vi "Backpropagation.vi"(8 "All Inputs":T2[](array[typedef]), 9 "Derrivatives":T2[](array[typedef]), 10 "Error":dbl[](array[numeric]), 11 "Neural Network In":refnum<class "Neural Network.lvclass">) -> (1 "Gradient Out":T1[](array[typedef]))   [LabVIEW 2015, in "Neural Network.lvclass"]
uses:
  Neural Network.lvclass
  Types/2D Array.ctl
  <vilib>/Analysis/NI_AALBase.lvlib
  <vilib>/Analysis/baseanly.llb/Real Outer Product.vi
  <vilib>/Analysis/Matrix/NI_Matrix.lvlib
  <vilib>/Analysis/Matrix/Numeric/Conversions/Matrix To Array - RM.vi
  Types/1D Array.ctl
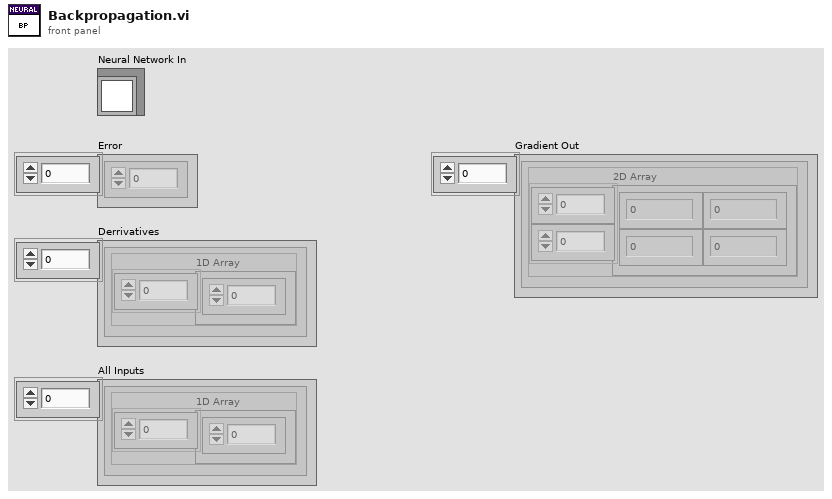
[diagram p1: front panel]
types:
  T1 = typedef "Neural Network.lvclass/2D Array.ctl" = cluster{"2D Array":sgl[][]}
  T2 = typedef "Neural Network.lvclass/1D Array.ctl" = cluster{"1D Array":dbl[]}
  T3 = typedef "NI_Matrix.lvlib/RealMatrix.ctl" = dbl[][]
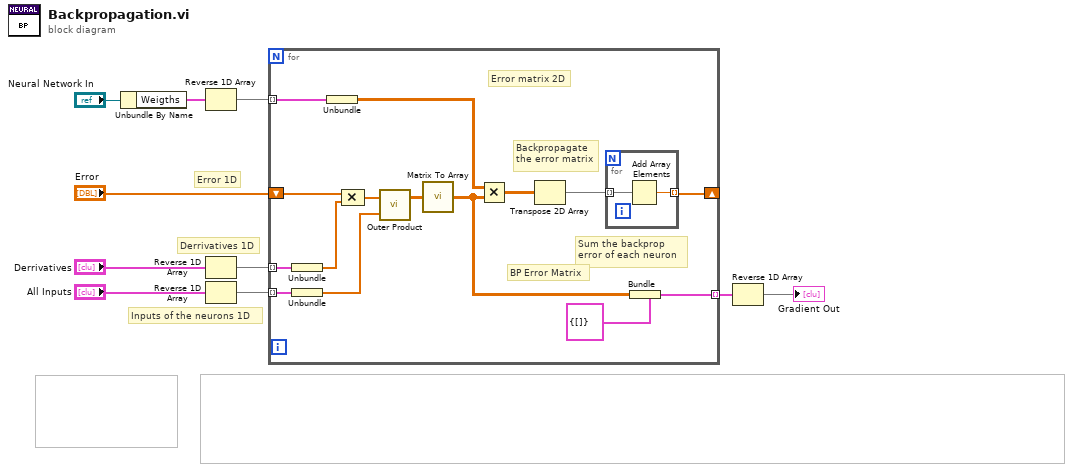
[diagram p0: block diagram]
diagram:
  # "Error 1D"
  # "Inputs of the neurons 1D"
  # "Derrivatives 1D"
  n1 = Unbundle By Name("Neural Network In") -> ("Weigths"=w1:T1[])
  n2 = Reverse 1D Array(array=w1) -> (reversed array=w9:T1[])
  n3 = Reverse 1D Array(array="Derrivatives") -> (reversed array=w7:T2[])
  n4 = Reverse 1D Array(array="All Inputs") -> (reversed array=w8:T2[])
  n5 = for {
    tunnel: w7 -> [w25] mode=indexing
    tunnel: w8 -> [w24] mode=indexing
    tunnel: w9 -> [w18] mode=indexing
    shift-right: [w22] -> _
    shift-left: "Error" -> [w20]
    tunnel: [w21] -> w10 mode=indexing
    # "BP Error Matrix"
    # "Sum the backprop\nerror of each neuron"
    # "Backpropagate\nthe error matrix"
    # "Error matrix 2D"
    n6 = Unbundle(w25) -> ("1D Array"=w23:dbl[])
    n7 = Unbundle(w24) -> ("1D Array"=w15:dbl[])
    n8 = Unbundle(w18) -> ("2D Array"=w13:sgl[][])
    n9 = Compound Arithmetic op=MULTIPLY(w20, w23) -> (w16:dbl[])
    n10 = call-poly <vilib>:"Outer Product.vi"("Y Vector"=w15, "X Vector"=w16) -> ("Outer Product"=w14:T3)  [unwired: 1 out]
    n11 = call-poly <vilib>:"Matrix To Array.vi"("Real Matrix"=w14) -> ("Real 2D Array"=w11:dbl[][])
    n12 = Multiply ("Multiply.vi")(x=w13, y=w11) -> (x*y=w12:dbl[][])
    n13 = Transpose 2D Array(2D array=w12) -> (transposed array=w17:dbl[][])
    n14 = for {
      tunnel: w17 -> [w27] mode=indexing
      tunnel: [w26] -> w22 mode=indexing
      n15 = Add Array Elements(numeric array=w27) -> (sum=w26:dbl)
    }
    n16 = Bundle(cluster=T1 {"2D Array"=[]}, "2D Array"=w11) -> (w21:T1)
  }
  n17 = Reverse 1D Array(array=w10) -> (reversed array=→"Gradient Out":T1[])
